vi "Send UDP Message.vi"(5 "Remote UDP Listening Port":u16, 7 "Remote IP":string, 8 "error in":errorcluster, 10 "UDP Data to be sent":string, 11 "Local UDP connection ref":refnum<k16>) -> (0 "error out":errorcluster, 3 "Local UDP connection ref out":refnum<k16>)   [LabVIEW 2021, in "UDP Comms.lvlib"]
uses:
  UDP Comms.lvlib
panel:
  in  "Timeout (ms)":i32
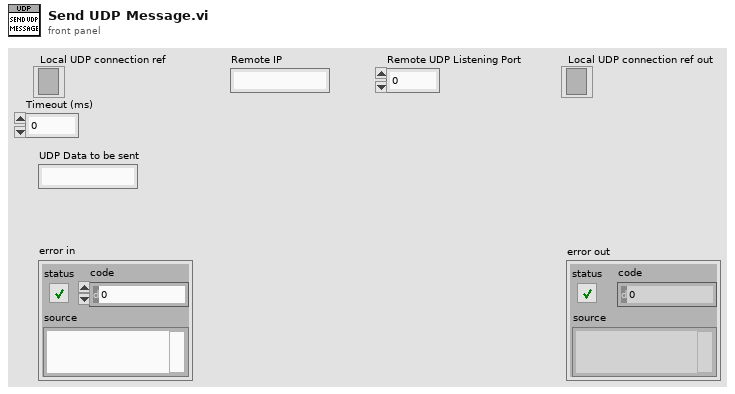
[diagram p1: front panel]
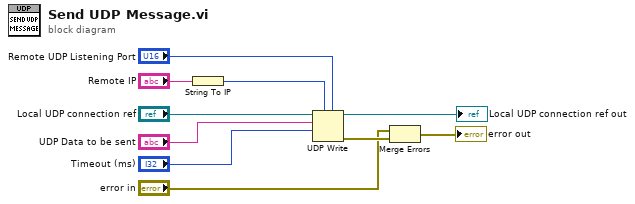
[diagram p0: block diagram]
diagram:
  n1 = String To IP(1:"Remote IP") -> (0:w10:u32)
  n2 = UDP Write(address=w10, port or service name="Remote UDP Listening Port", connection ID="Local UDP connection ref", data in="UDP Data to be sent", 9:"Timeout (ms)") -> (error out=w4:errorcluster, 3:→"Local UDP connection ref out":refnum<k16>)  [unwired: 1 in]
  n3 = Merge Errors("error in", w4) -> (→"error out":errorcluster)
